vi "GetPointType4D_2D-SGL.vi"(11 "Point":T2) -> (3 "Point":T1)   [LabVIEW 2020, in "OpenLvVision_OpenCv.lvlib"]
uses:
  OpenLvVision_OpenCv.lvlib
  TypeDef/Point/4D_PointSGL.ctl
  TypeDef/Point/2D_PointSGL.ctl
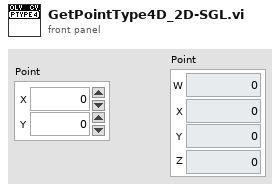
[diagram p1: front panel]
types:
  T1 = typedef "OpenLvVision_OpenCv.lvlib/4D_PointSGL.ctl" = cluster{"W":sgl, "X":sgl, "Y":sgl, "Z":sgl}
  T2 = typedef "OpenLvVision_OpenCv.lvlib/2D_PointSGL.ctl" = cluster{"X":sgl, "Y":sgl}
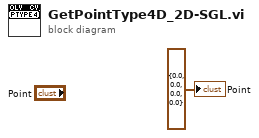
[diagram p0: block diagram]
diagram:
  "Point" <- T1 {"W"=0.0, "X"=0.0, "Y"=0.0, "Z"=0.0} ("Point")
